vi "joystick interface.vi"() -> ()   [LabVIEW 2009]
uses:
  crabe drive.ctl
panel:
  out "output":T1 {"turn" scale=-1.0..1.0; "skew (direction)" scale=0.0..6.28318470517958 scale format="%.1g"; "speed" scale=-1.0..1.0}
  in  "footpedal":cluster{"speed":dbl, "direction":bool}={"speed"=0.0, "direction"=TRUE} {"speed" scale=0.0..1.0}
  in  "joystick":cluster{"y":dbl, "x":dbl, "turn":dbl} {"turn" scale=-1.0..1.0; "x" scale=-1.0..1.0; "y" scale=-1.0..1.0}
  # "fwd"
  # "rev"
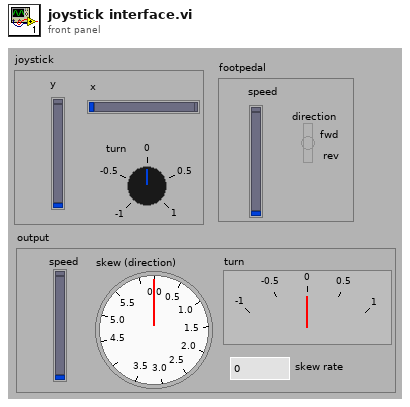
[diagram p1: front panel]
types:
  T1 = typedef "crabe drive.ctl" = cluster{"speed":dbl, "skew (direction)":dbl, "turn":dbl, "skew rate":dbl}
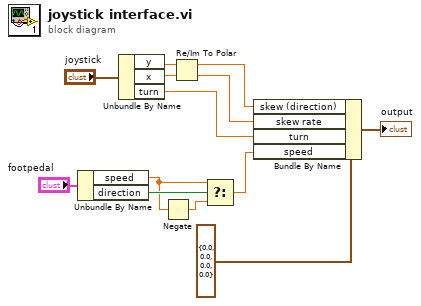
[diagram p0: block diagram]
diagram:
  n1 = Unbundle By Name("footpedal") -> ("speed"=w9:dbl, "direction"=w12:bool)
  n2 = Unbundle By Name("joystick") -> ("y"=w8:dbl, "x"=w7:dbl, "turn"=w2:dbl)
  n3 = Negate(x=w9) -> (-x=w11:dbl)
  n4 = Re/Im To Polar(2:w7, 3:w8) -> (0:w3:dbl, 1:w4:dbl)
  n5 = Select(t=w9, s=w12, f=w11) -> (s? t:f=w5:dbl)
  n6 = Bundle By Name(cluster=T1 {"speed"=0.0, "skew (direction)"=0.0, "turn"=0.0, "skew rate"=0.0} ("output"), "skew (direction)"=w4, "skew rate"=w3, "turn"=w2, "speed"=w5) -> (→"output":T1)
